vi "Config Aout CFactor.vi"(8 "error in":errorcluster, 9 "Loss (100.0 V/pF)":dbl=100.0 min=-999999999.9 max=99999999.8 format="%#_9f", 10 "Capacitance (10.0 V/pF)":dbl=10.0 min=-999999999.9 max=99999999.8 format="%#_9f", 11 "VISA resource name":refnum<visa-resource-name>) -> (0 "error out":errorcluster, 3 "VISA resource name out":refnum<visa-resource-name>)   [LabVIEW 2017, in "Andeen-Hagerling 2700.lvlib"]
doc: "This VI sets the input to output voltage conversion factor for the capacitance and loss voltage output channels in V/pF and V/jpF respectively. This command gives a direct means of controlling the sensitivity of the voltage outputs to changes in the DUT."
uses:
  Andeen-Hagerling 2700.lvlib
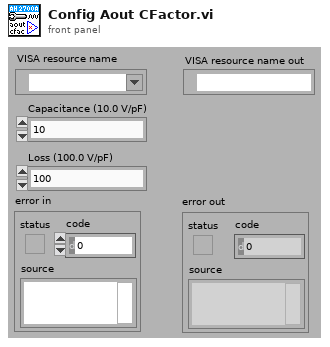
[diagram p1: front panel]
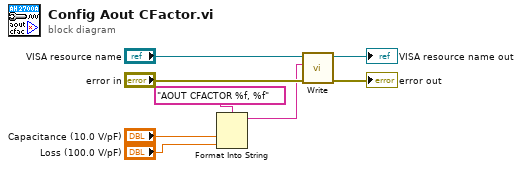
[diagram p0: block diagram]
diagram:
  n1 = Format Into String(format string="AOUT CFACTOR %f, %f", "Capacitance (10.0 V/pF)", "Loss (100.0 V/pF)") -> (resulting string=w1:string)  [unwired: 2 in, 1 out]
  n2 = call "Write.vi"("error in"="error in", "command"=w1, "VISA resource name"="VISA resource name") -> ("error out"=→"error out":errorcluster, "VISA resource name out"=→"VISA resource name out":refnum<visa-resource-name>)  [unwired: 7 in]
